vi "output.vi"(8 "error in (no error)":errorcluster, 10 "Output [on/off]":bool, 11 "PSP-603 in":refnum<class "PSP-603.lvclass">) -> (0 "error out":errorcluster, 3 "PSP-603 out":refnum<class "PSP-603.lvclass">)   [LabVIEW 2025, in "Power Supply.lvlib" / "PSP-603.lvclass"]
uses:
  PSP-603.lvclass
  PSP-603.lvclass/PSP-603.ctl
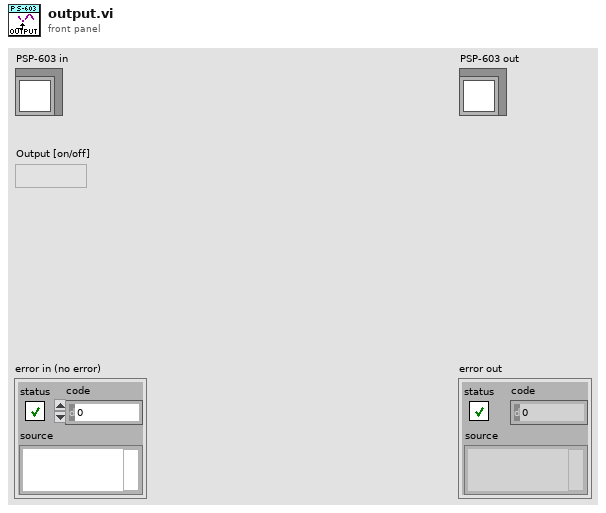
[diagram p1: front panel]
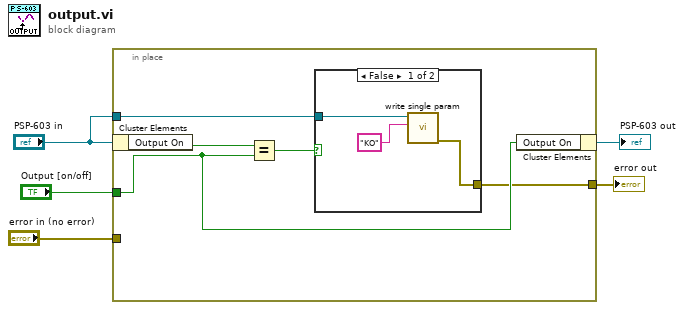
[diagram p0: block diagram]
diagram:
  n1 = in-place {
    in-place-border: "Output [on/off]" -> [w9]
    in-place-border: "PSP-603 in" -> [w7]
    in-place-border: [w6] -> w2
    in-place-border: "error in (no error)" -> [_]
    n2 = in-place-cluster #1("PSP-603 in") -> ("Output On"=w10:bool)
    n3 = Equal?(x=w10, y=w9) -> (x = y?=w8:bool)
    n4 = case shown="False" w8 {
      tunnel: w7 -> [w13 _]
      tunnel: [w11 _] -> w6
      frame False {
        n5 = call-dynamic "write single param.vi"("string"="KO", "PSP-603 in"=w13) -> ("error out"=w11:errorcluster)  [unwired: 8 in, 1 out]
      }
      frame True {
      }
    }
    n6 = in-place-cluster #1("Output On"=w9) -> (→"PSP-603 out":refnum<class "PSP-603.lvclass">)
  }
  "error out" <- w2
